vi "Trace Message.vi"(8 "error in (no error)":errorcluster, 10 "Message":string, 11 "Tracer-P in":refnum<class "Tracer-P.lvclass">) -> (0 "error out":errorcluster, 3 "Tracer-P out":refnum<class "Tracer-P.lvclass">)   [LabVIEW 2013, in "Tracer-P.lvclass"]
uses:
  Tracer-P.lvclass
  Logical Systems/Tracer/Tracer.lvclass
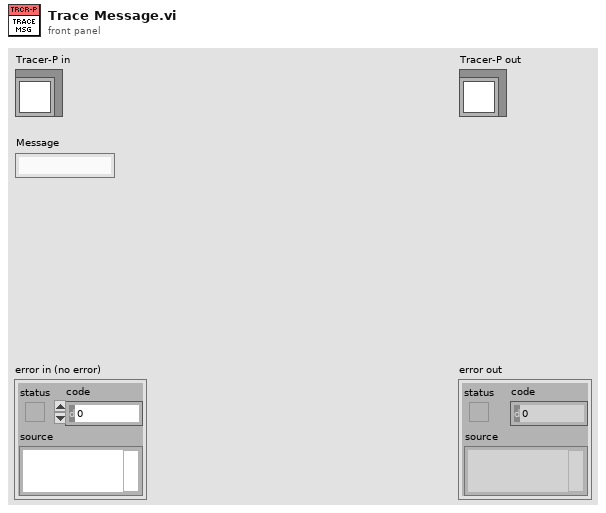
[diagram p1: front panel]
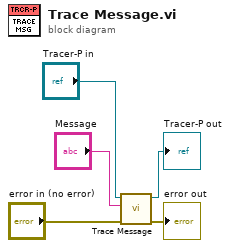
[diagram p0: block diagram]
diagram:
  n1 = call-parent "Trace Message.vi"("error in (no error)"="error in (no error)", "Message"="Message", "System in"="Tracer-P in") -> ("error out"=→"error out":errorcluster, "System out"=→"Tracer-P out":refnum<class "Tracer-P.lvclass">)  [unwired: 7 in]
